vi "sub_xygraph.vi"(11 "wf":waveform(dbl)[](array[waveform])) -> (2 "xy-limit":cluster{dbl[], dbl[]}[](array[cluster]), 3 "xy_data":cluster{dbl[], dbl[]}, 5 "xy_out":cluster{dbl, dbl}[](array[cluster]))   [LabVIEW 2013]
uses:
  <vilib>/measure/madcrms.llb/Basic Averaged DC-RMS for 1 Chan.vi
  <vilib>/measure/NI_MAPro.lvlib
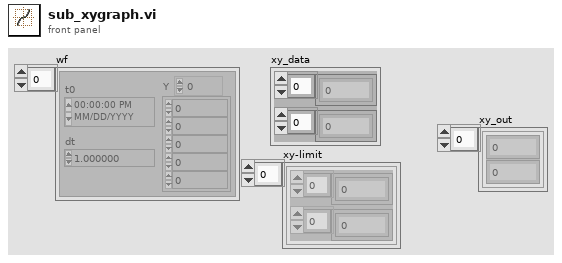
[diagram p1: front panel]
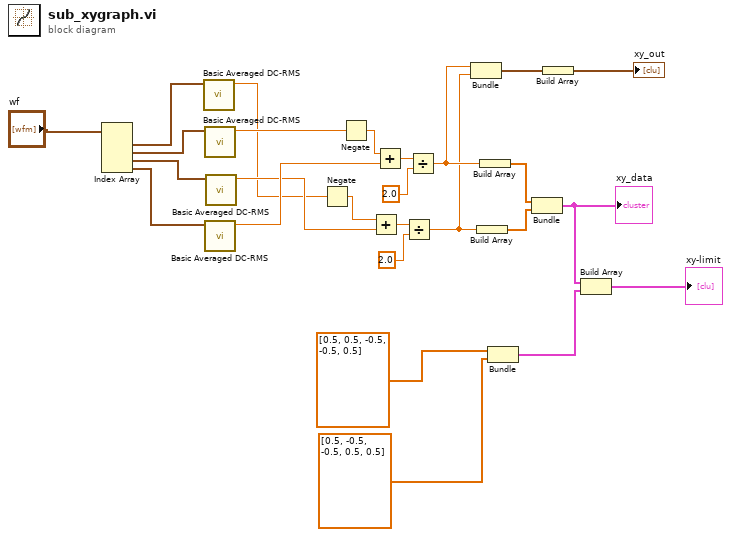
[diagram p0: block diagram]
diagram:
  n1 = Index Array(array="wf") -> (element #1=w19:waveform(dbl), element #2=w20:waveform(dbl), element #3=w21:waveform(dbl), element #4=w22:waveform(dbl))  [unwired: 4 in]
  n2 = call-poly <vilib>:"Basic Averaged DC-RMS.vi"("signal in"=w19) -> ("DC value"=w23:dbl)  [unwired: 7 in, 3 out]
  n3 = call-poly <vilib>:"Basic Averaged DC-RMS.vi"("signal in"=w20) -> ("DC value"=w24:dbl)  [unwired: 7 in, 3 out]
  n4 = call-poly <vilib>:"Basic Averaged DC-RMS.vi"("signal in"=w22) -> ("DC value"=w26:dbl)  [unwired: 7 in, 3 out]
  n5 = call-poly <vilib>:"Basic Averaged DC-RMS.vi"("signal in"=w21) -> ("DC value"=w25:dbl)  [unwired: 7 in, 3 out]
  n6 = Negate(x=w23) -> (-x=w18:dbl)
  n7 = Negate(x=w24) -> (-x=w17:dbl)
  n8 = Add(x=w18, y=w25) -> (x+y=w12:dbl)
  n9 = Add(x=w17, y=w26) -> (x+y=w14:dbl)
  n10 = Divide(x=w12, y=2.0) -> (x/y=w3:dbl)
  n11 = Divide(x=w14, y=2.0) -> (x/y=w4:dbl)
  n12 = Bundle(w4, w3) -> (w2:cluster{dbl, dbl})  [unwired: 1 in]
  n13 = Build Array(w3) -> (w5:dbl[])
  n14 = Build Array(w4) -> (w6:dbl[])
  n15 = Bundle(dbl[] [0.5, 0.5, -0.5, -0.5, 0.5], dbl[] [0.5, -0.5, -0.5, 0.5, 0.5]) -> (w9:cluster{dbl[], dbl[]})  [unwired: 1 in]
  n16 = Bundle(w6, w5) -> (w7:cluster{dbl[], dbl[]})  [unwired: 1 in]
  "xy_data" <- w7
  n17 = Build Array(w2) -> (→"xy_out":cluster{dbl, dbl}[])
  n18 = Build Array(w7, w9) -> (→"xy-limit":cluster{dbl[], dbl[]}[])
